vi "Open DSF Configuration Data.vi"(8 "error in (no error)":errorcluster, 9 "replace if found? (F)":bool, 10 "create file if necessary (T)":bool=TRUE, 11 "dsf configuration file path":path) -> (0 "error out":errorcluster, 1 "file replaced?":bool, 2 "file created?":bool, 3 "dsf refnum":T2, 4 "version":T1)   [LabVIEW 2017, in "DSF Configuration API.lvlib"]
doc: "Opens a reference to the configuration data found in a platform-independent configuration file."
uses:
  DSF Configuration API.lvlib
  Controls/DSF Config Data RefNum.ctl
  Controls/DSF Version Info.ctl
  Private/Controls/Session/DSF Config Data.ctl
  Private/Controls/DSF File Format/Internal.DSF Configuration.ctl
  Private/Controls/DSF File Format/Internal.DSF Plugin with ID.ctl
  Private/Controls/DSF File Format/Internal.DSF Plugin Info.ctl
  Controls/DSF Timing Info.ctl
  Private/Controls/DSF File Format/Internal.DSF Group with ID.ctl
  Private/Controls/DSF File Format/Internal.DSF Group Info.ctl
  Private/Controls/DSF File Format/Internal.DSF Transfer with ID.ctl
  Private/Controls/DSF File Format/Internal.DSF Transfer Info.ctl
  Private/Controls/DSF File Format/Internal.DSF Channel with ID.ctl
  Private/Controls/DSF File Format/Internal.DSF Channel Info.ctl
  Private/Controls/DSF File Format/Internal.DSF Settings with ID.ctl
  Private/Controls/DSF File Format/Internal.DSF Settings Info.ctl
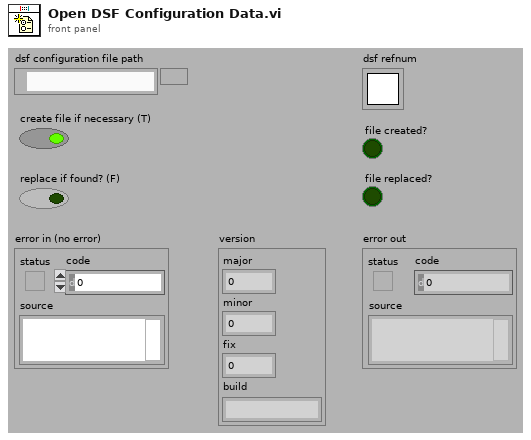
[diagram p1: front panel]
types:
  T1 = typedef "DSF Configuration API.lvlib/DSF Version Info.ctl" = cluster{"major":u32, "minor":u32, "fix":u32, "build":string}
  T2 = typedef "DSF Configuration API.lvlib/DSF Config Data RefNum.ctl" = refnum<k1>
  T3 = typedef "DSF Configuration API.lvlib/DSF Config Data.ctl" = cluster{"dsf configuration":T4, "path":path, "dirty":bool}
  T4 = typedef "DSF Configuration API.lvlib/Internal.DSF Configuration.ctl" = cluster{"dsfversion":T1, "version":T1, "plugins":T5[], "groups":T8[], "transfers":T10[], "channels":T12[], "settings":T14[]}
  T5 = typedef "DSF Configuration API.lvlib/Internal.DSF Plugin with ID.ctl" = cluster{"id":string, "values":T6}
  T6 = typedef "DSF Configuration API.lvlib/Internal.DSF Plugin Info.ctl" = cluster{"type":string, "timing":T7, "group ids":string[], "settings id":string}
  T7 = typedef "DSF Configuration API.lvlib/DSF Timing Info.ctl" = cluster{"priority":u64, "decimation":u64, "offset":u64}
  T8 = typedef "DSF Configuration API.lvlib/Internal.DSF Group with ID.ctl" = cluster{"id":string, "values":T9}
  T9 = typedef "DSF Configuration API.lvlib/Internal.DSF Group Info.ctl" = cluster{"direction":i32, "timing":T7, "transfer ids":string[], "settings id":string}
  T10 = typedef "DSF Configuration API.lvlib/Internal.DSF Transfer with ID.ctl" = cluster{"id":string, "values":T11}
  T11 = typedef "DSF Configuration API.lvlib/Internal.DSF Transfer Info.ctl" = cluster{"byte order":i32, "channel ids":string[], "settings id":string}
  T12 = typedef "DSF Configuration API.lvlib/Internal.DSF Channel with ID.ctl" = cluster{"id":string, "values":T13}
  T13 = typedef "DSF Configuration API.lvlib/Internal.DSF Channel Info.ctl" = cluster{"count":u64, "buffer offset":u64, "data type":i32, "settings id":string}
  T14 = typedef "DSF Configuration API.lvlib/Internal.DSF Settings with ID.ctl" = cluster{"id":string, "values":T15}
  T15 = typedef "DSF Configuration API.lvlib/Internal.DSF Settings Info.ctl" = cluster{"key":string, "value":string}[]
  T16 = typedef "DSF Configuration API.lvlib/DSF Configuration Reference.ctl" = refnum<data-value>
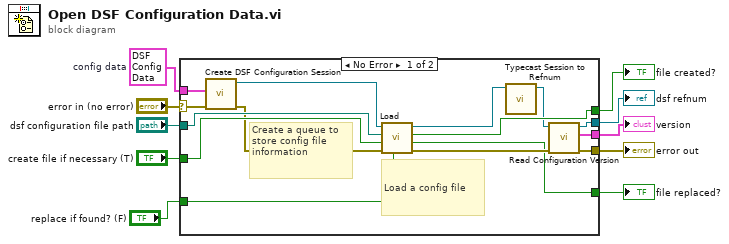
[diagram p0: block diagram]
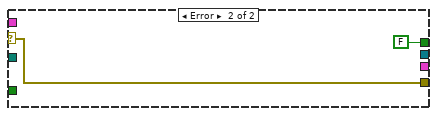
[diagram p2: hidden frame]
diagram:
  w4 = T3 {"dsf configuration"={"dsfversion"={"major"=0, "minor"=0, "fix"=0, "build"=""}, "version"={"major"=0, "minor"=0, "fix"=0, "build"=""}, "plugins"=[], "groups"=[], "transfers"=[], "channels"=[], "settings"=[]}, "path"=path "", "dirty"=FALSE}  # config data
  n1 = case shown="No Error" "error in (no error)" {
    selector: "error in (no error)" -> [w21 w27]
    tunnel: "dsf configuration file path" -> [w25 _]
    tunnel: "create file if necessary (T)" -> [w24 _]
    tunnel: [w22 FALSE ("file created?")] -> w6
    tunnel: [w17 w27] -> w7
    tunnel: w4 -> [w13 _]
    tunnel: [w15 _] -> w5
    tunnel: [w14 _] -> w3
    tunnel: "replace if found? (F)" -> [w12 _]
    tunnel: [w11 _] -> w1
    frame No Error {
      # "Load a config file"
      # "Create a queue to store config file information"
      n2 = call "Create DSF Configuration Session.vi"("error in (no error)"=w21, "config data"=w13) -> ("error out"=w20:errorcluster, "DSF Configuration Session out"=w18:T16)  [unwired: 8 in]
      n3 = call "Load.vi"("replace if found? (F)"=w12, "error in (no error)"=w20, "create file if necessary? (T)"=w24, "configuration file path"=w25, "DSF Configuration Reference in"=w18) -> ("error out"=w23:errorcluster, "file replaced?"=w11:bool, "file created?"=w22:bool, "DSF Configuration Reference out"=w19:T16)  [unwired: 3 out]
      n4 = call "Typecast Session to Refnum.vi"("DSF Configuration Session in"=w19) -> ("dsf refnum out"=w16:T2)  [unwired: 10 in]
      n5 = call "Read Configuration Version.vi"("error in (no error)"=w23, "dsf refnum"=w16) -> ("error out"=w17:errorcluster, "version"=w14:T1, "dsf refnum out"=w15:T2)  [unwired: 7 in]
    }
    frame Error {
    }
  }
  "error out" <- w7
  "file created?" <- w6
  "dsf refnum" <- w5
  "version" <- w3
  "file replaced?" <- w1
